vi "ScriptedStateMachine.vi"(8 "ErrorArray":errorcluster[](array[cluster]), 10 "Script":string[](array[string]), 11 "TestBase.lvclass":refnum<class "TestBase.lvclass">) -> (0 "ErrorArray":errorcluster[](array[cluster]), 2 "Data":variant, 3 "TestBase.lvclass":refnum<class "TestBase.lvclass">)   [LabVIEW 2014, in "TestBase.lvclass"]
uses:
  TestBase.lvclass
  TestBase.lvclass/TestBase.ctl
  Accessors/Read ErrorSeverity.vi
  <vilib>/Utility/error.llb/Error Cluster From Error Code.vi
  <vilib>/ErrorRing/Error Ring.xnode
  <userlib>/NIST/NISTErrorLib/NISTErrorLib.lvlib
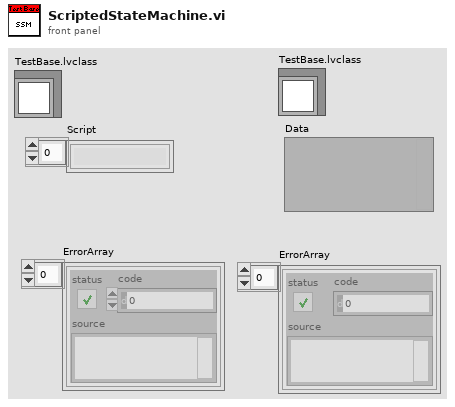
[diagram p1: front panel]
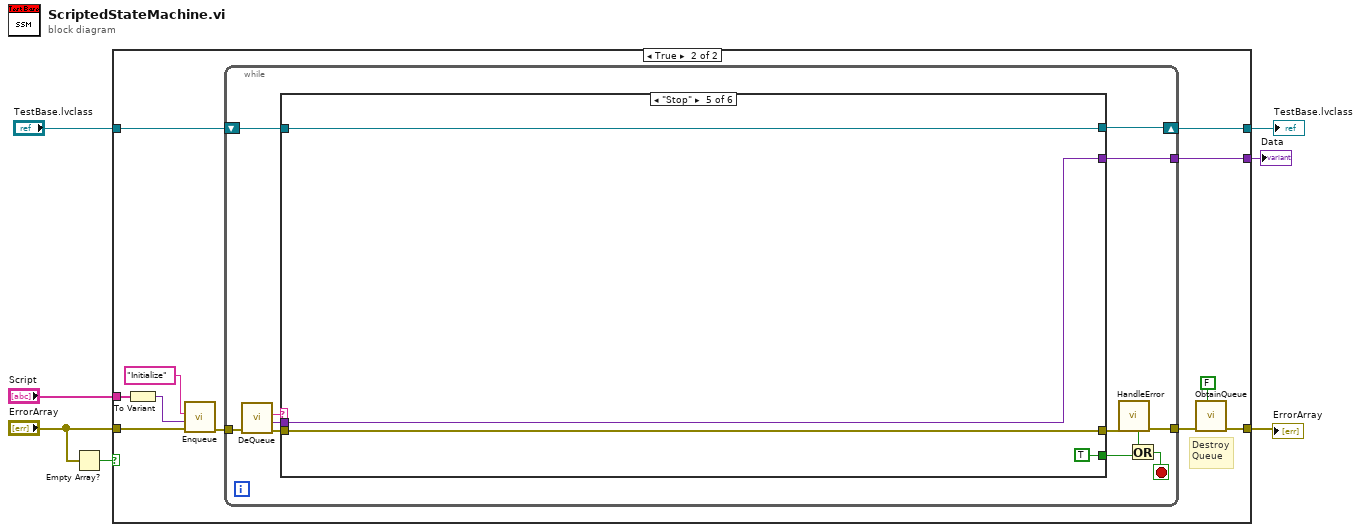
[diagram p0: block diagram]
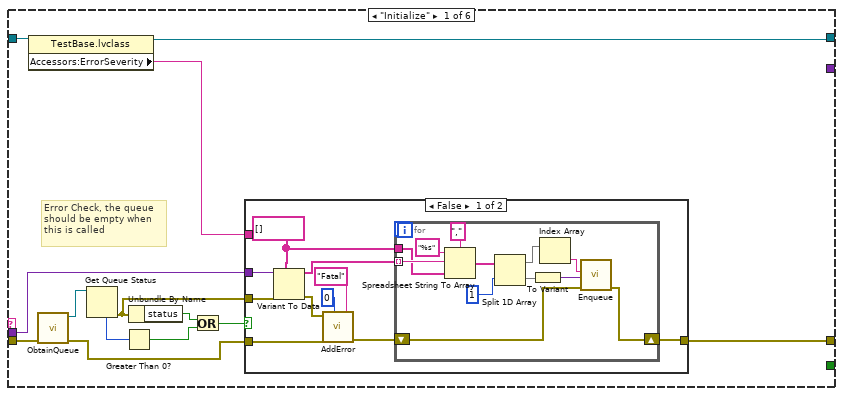
[diagram p3: hidden frame]
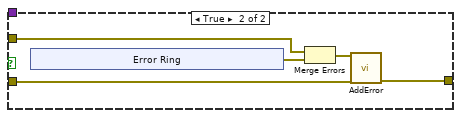
[diagram p4: hidden frame]
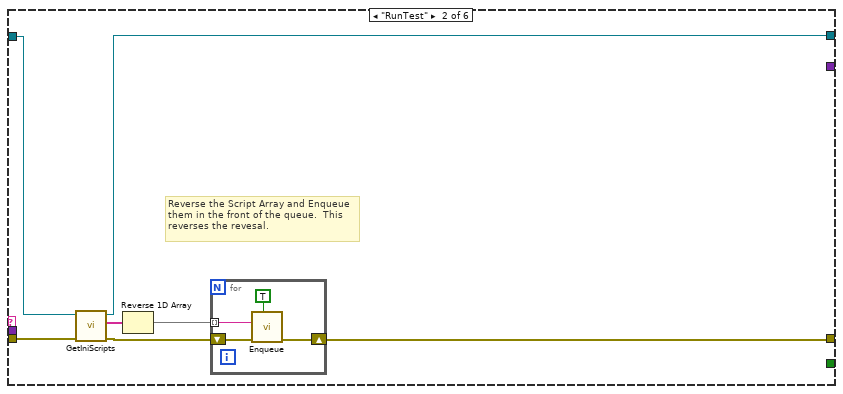
[diagram p5: hidden frame]
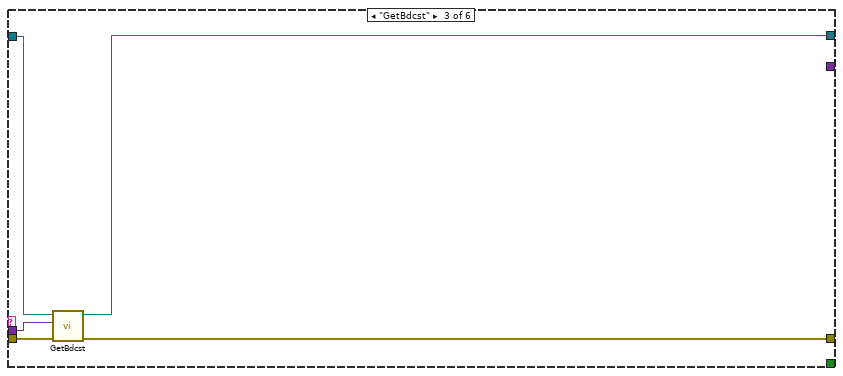
[diagram p6: hidden frame]
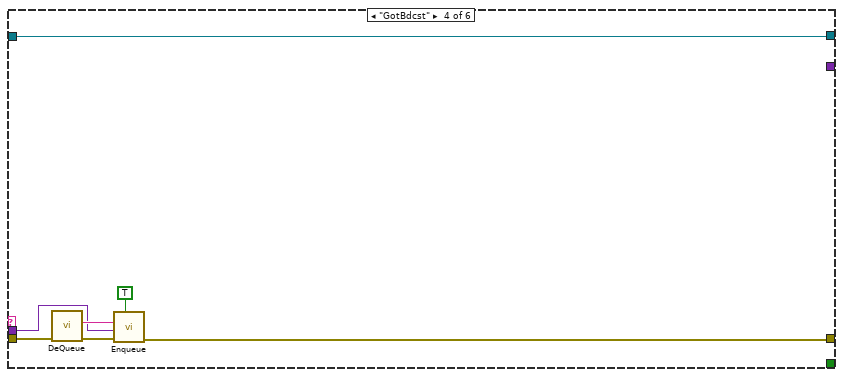
[diagram p7: hidden frame]
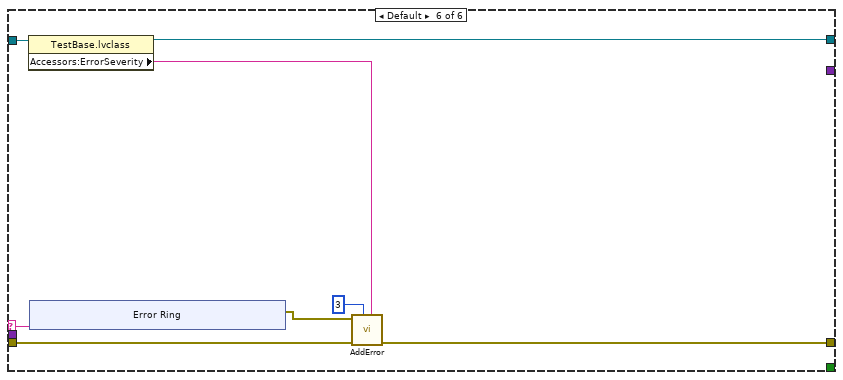
[diagram p8: hidden frame]
diagram:
  n1 = Empty Array?(array="ErrorArray") -> (empty?=w6:bool)
  n2 = case shown="True" w6 {
    tunnel: "ErrorArray" -> [w8 w19]
    tunnel: [w9 w11] -> w4
    tunnel: "TestBase.lvclass" -> [w9 w12]
    tunnel: [w8 w16] -> w3
    tunnel: "Script" -> [_ w20]
    tunnel: [_ w10] -> w1
    frame False {
    }
    frame True {
      # "Destroy\nQueue"
      n3 = To Variant(anything=w20) -> (Variant=w18:variant)
      n4 = call "Enqueue.vi"("ErrorArray"=w19, "Data"=w18, "Message"="Initialize") -> ("ErrorArray"=w13:errorcluster[])  [unwired: 8 in]
      n5 = while {
        tunnel: [w32] -> w14
        tunnel: w13 -> [w31]
        shift-right: [w26] -> w11
        shift-left: w12 -> [w27]
        tunnel: [w21] -> w10
        stop <- w22 stop-if-true
        n6 = call "DeQueue.vi"("ErrorArray"=w31) -> ("ErrorArray"=w28:errorcluster[], "Data"=w29:variant, "Message"=w30:string)  [unwired: 8 in]
        n7 = case shown="\"Stop\"" w30 {
          selector: w30 -> [_ _ _ _ _ w112]
          tunnel: w29 -> [w35 _ w92 w96 w101 _]
          tunnel: w28 -> [w45 w84 w93 w100 w102 w111]
          tunnel: w27 -> [w38 w83 w91 w94 w103 w108]
          tunnel: [w33 w81 w90 w94 w103 w106] -> w26
          tunnel: [w34 w78 w89 w95 w102 w105] -> w25
          tunnel: [_ _ _ _ TRUE _] -> w23
          tunnel: [_ _ _ _ w101 _] -> w21
          frame "Initialize" {
            # "Error Check, the queue\nshould be empty when\nthis is called"
            n8 = property class="TestBase.lvclass"(reference=w38) -> (reference out=w33:refnum<class "TestBase.lvclass">, "Accessors:ErrorSeverity"=w37:string)  [unwired: 1 in, 1 out]
            n9 = call "ObtainQueue.vi"("ErrorArray"=w45) -> ("ErrorArray."=w36:errorcluster[], "TstQue"=w44:refnum<queue>)  [unwired: 9 in]
            n10 = Get Queue Status(queue=w44) -> (error out=w39:errorcluster, # elements in queue=w43:i32)  [unwired: 2 in, 6 out]
            n11 = Greater Than 0?(x=w43) -> (x > 0?=w41:bool)
            n12 = Unbundle By Name(w39) -> ("status"=w42:bool)
            n13 = Or(x=w42, y=w41) -> (x .or. y?=w40:bool)
            n14 = case shown="False" w40 {
              tunnel: w39 -> [w54 w71]
              tunnel: w37 -> [_ _]
              tunnel: w36 -> [w52 w69]
              tunnel: [w46 w68] -> w34
              tunnel: w35 -> [w55 _]
              frame False {
                w47 = string[] []
                n15 = Variant To Data(error in=w54, type=w47, Variant=w55) -> (data=w48:string[], error out=w53:errorcluster)
                n16 = call <userlib>:"AddError.vi"("Severity"="Fatal", "Priority"=u8 0, "ErrorArray"=w52, "error in (no error)"=w53) -> ("ErrorArray"=w49:errorcluster[])  [unwired: 6 in, 1 out]
                n17 = for {
                  shift-right: [w56] -> w46
                  shift-left: w49 -> [w57]
                  tunnel: w48 -> [w67] mode=indexing
                  tunnel: w47 -> [w64]
                  n18 = Spreadsheet String To Array(delimiter (Tab)=",", format string="%s", spreadsheet string=w67, array type (2D Dbl)=w64) -> (array=w63:string[])
                  n19 = Split 1D Array(array=w63, index=1) -> (first subarray=w61:string[], second subarray=w60:string[])
                  n20 = To Variant(anything=w60) -> (Variant=w58:variant)
                  n21 = Index Array(array=w61) -> (element=w59:string)  [unwired: 1 in]
                  n22 = call "Enqueue.vi"("ErrorArray"=w57, "Data"=w58, "Message"=w59) -> ("ErrorArray"=w56:errorcluster[])  [unwired: 8 in]
                }
              }
              frame True {
                n23 = xnode "Error Ring"() -> ("error out"=w72:errorcluster)
                n24 = Merge Errors(w71, w72) -> (w70:errorcluster)
                n25 = call <userlib>:"AddError.vi"("ErrorArray"=w69, "error in (no error)"=w70) -> ("ErrorArray"=w68:errorcluster[])  [unwired: 8 in, 1 out]
              }
            }
          }
          frame "RunTest" {
            # "Reverse the Script Array and Enqueue them in the front of the queue.  This reverses the revesal."
            n26 = call "GetIniScripts.vi"("ErrorArray"=w84, "TestBase.lvclass"=w83) -> ("ErrorArray"=w80:errorcluster[], "Script"=w82:string[], "TestBase.lvclass"=w81:refnum<class "TestBase.lvclass">)  [unwired: 7 in]
            n27 = Reverse 1D Array(array=w82) -> (reversed array=w79:string[])
            n28 = for {
              shift-right: [w87] -> w78
              shift-left: w80 -> [w88]
              tunnel: w79 -> [w85] mode=indexing
              n29 = call "Enqueue.vi"("Priority(?) (f)"=TRUE, "ErrorArray"=w88, "Message"=w85) -> ("ErrorArray"=w87:errorcluster[])  [unwired: 8 in]
            }
          }
          frame "GetBdcst" {
            n30 = call "GetBdcst.vi"("ErrorArray"=w93, "BdcstInfo"=w92, "TestBase.lvclass"=w91) -> ("ErrorArray"=w89:errorcluster[], "TestBase.lvclass"=w90:refnum<class "TestBase.lvclass">)  [unwired: 7 in]
          }
          frame "GotBdcst" {
            n31 = call "DeQueue.vi"("ErrorArray"=w100) -> ("ErrorArray"=w99:errorcluster[], "Message"=w97:string)  [unwired: 8 in, 1 out]
            n32 = call "Enqueue.vi"("Priority(?) (f)"=TRUE, "ErrorArray"=w99, "Data"=w96, "Message"=w97) -> ("ErrorArray"=w95:errorcluster[])  [unwired: 7 in]
          }
          frame "Stop" {
          }
          frame Default {
            n33 = property class="TestBase.lvclass"(reference=w108) -> (reference out=w106:refnum<class "TestBase.lvclass">, "Accessors:ErrorSeverity"=w107:string)  [unwired: 1 in, 1 out]
            n34 = xnode "Error Ring"("parameter 0"=w112) -> ("error out"=w110:errorcluster)
            n35 = call <userlib>:"AddError.vi"("Severity"=w107, "Priority"=u8 3, "ErrorArray"=w111, "error in (no error)"=w110) -> ("ErrorArray"=w105:errorcluster[])  [unwired: 6 in, 1 out]
          }
        }
        n36 = call "HandleError.vi"("ErrorArray"=w25) -> ("ErrorArray"=w32:errorcluster[], "Stop"=w24:bool)  [unwired: 9 in]
        n37 = Or(x=w24, y=w23) -> (x .or. y?=w22:bool)
      }
      n38 = call "ObtainQueue.vi"("Destroy? (f)"=FALSE, "ErrorArray"=w14) -> ("ErrorArray."=w16:errorcluster[])  [unwired: 8 in, 1 out]
    }
  }
  "TestBase.lvclass" <- w4
  "ErrorArray" <- w3
  "Data" <- w1
